vi "Read Voltage.vi"(8 "error in (no error)":errorcluster, 11 "Update Fan Voltage MSG in":refnum<class "Update Fan Voltage MSG.lvclass">) -> (0 "error out":errorcluster, 2 "Voltage":dbl, 3 "Update Fan Voltage MSG out":refnum<class "Update Fan Voltage MSG.lvclass">)   [LabVIEW 2016, in "Controller.lvlib" / "Update Fan Voltage MSG.lvclass"]
uses:
  Update Fan Voltage MSG.lvclass
  Update Fan Voltage MSG.lvclass/Update Fan Voltage MSG.ctl
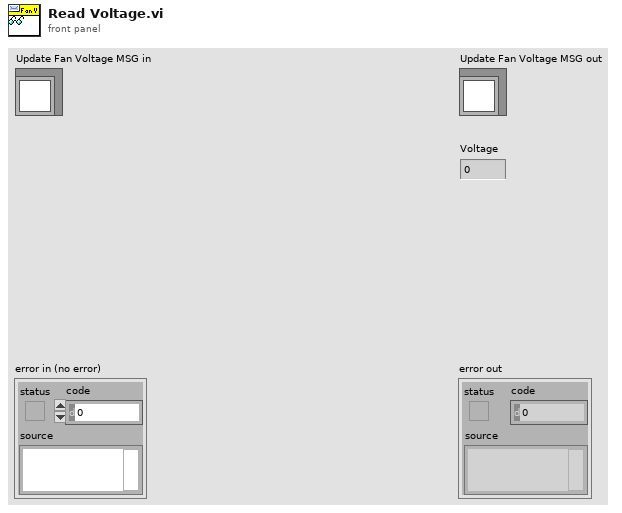
[diagram p1: front panel]
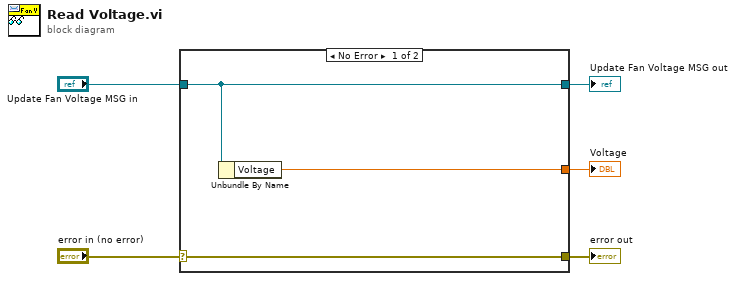
[diagram p0: block diagram]
diagram:
  n1 = case shown="No Error" "error in (no error)" {
    selector: "error in (no error)" -> [w8 w9]
    tunnel: [w8 w9] -> w4
    tunnel: [w7 w10] -> w2
    tunnel: "Update Fan Voltage MSG in" -> [w7 w10]
    tunnel: [w6 _] -> w1
    frame No Error {
      n2 = Unbundle By Name(w7) -> ("Voltage"=w6:dbl)
    }
    frame Error {
    }
  }
  "error out" <- w4
  "Update Fan Voltage MSG out" <- w2
  "Voltage" <- w1
